vi "AllOff.vi"(6 "Update?":bool, 8 "RightIn":dbl, 9 "LeftIn":dbl, 11 "ButtonIn":bool) -> (0 "RightOut":dbl, 1 "LeftOut":dbl, 3 "Compressor":bool)   [LabVIEW 2017]
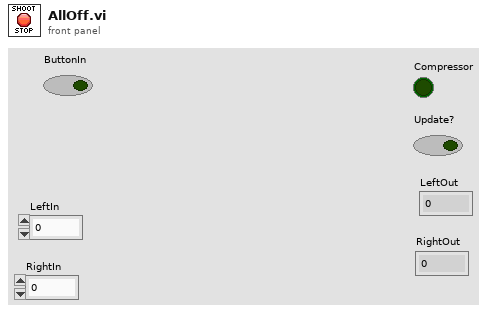
[diagram p1: front panel]
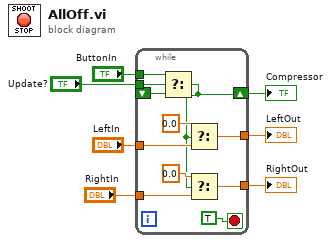
[diagram p0: block diagram]
diagram:
  n1 = while {
    tunnel: [w17] -> w7
    tunnel: [w16] -> w6
    tunnel: "RightIn" -> [w14]
    tunnel: "LeftIn" -> [w13]
    tunnel: "Update?" -> [w11]
    tunnel: "ButtonIn" -> [w10]
    shift-right: [w8] -> w1
    shift-left: _ -> [w9]
    stop <- TRUE stop-if-true
    n2 = Select(t=w10, s=w11, f=w9) -> (s? t:f=w8:bool)
    n3 = Select(t=0.0, s=w8, f=w13) -> (s? t:f=w17:dbl)
    n4 = Select(t=0.0, s=w8, f=w14) -> (s? t:f=w16:dbl)
  }
  "Compressor" <- w1
  "LeftOut" <- w7
  "RightOut" <- w6
